vi "macro_TrajectoryConstraint_SwerveKine.vi"   [LabVIEW 2019, in "Trajectory_Library.lvlib"]
uses:
  Trajectory_Library.lvlib
types:
  T1 = typedef "WPILib_Math.lvlib/TRANSLATION2D.ctl" = cluster{"X":dbl, "Y":dbl}
  T2 = typedef "WPILib_Math.lvlib/SWERVE_DRIVE_KINEMATICS.ctl" = cluster{"NumModules":i32, "InverseKinematics":T3, "ForwardKinematics":T3, "Modules":T1[], "PrevCoR":T1, "SavedModuleStates":T4[]}
  T3 = typedef "NI_Matrix.lvlib/RealMatrix.ctl" = dbl[][]
  T4 = typedef "WPILib_Math.lvlib/SWERVE_DRIVE_MODULE_STATE.ctl" = cluster{"Speed":dbl, "Angle":T5}
  T5 = typedef "WPILib_Math.lvlib/ROTATION2D.ctl" = cluster{"VALUE":dbl, "COS":dbl, "SIN":dbl}
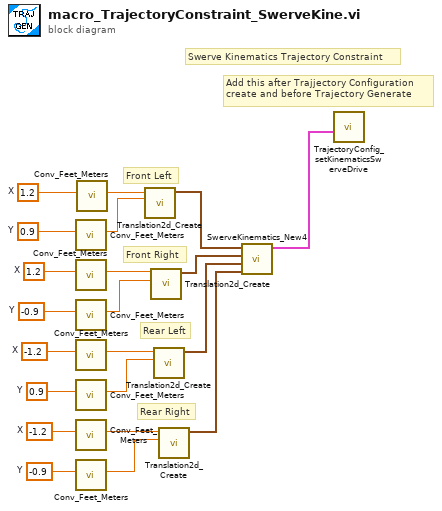
[diagram p0: block diagram]
diagram:
  w15 = -1.2  # X
  w14 = -0.9  # Y
  w17 = -1.2  # X
  w16 = 0.9  # Y
  w19 = 1.2  # X
  w18 = -0.9  # Y
  w21 = 1.2  # X
  w20 = 0.9  # Y
  # "Swerve Kinematics Trajectory Constraint"
  # "Rear Right"
  # "Rear Left"
  # "Front Right"
  # "Front Left"
  # "Add this after Trajjectory Configuration\ncreate and before Trajectory Generate"
  n1 = call "Conv_Feet_Meters.vi"("Feet"=w20) -> ("Meters"=w12:dbl)  [unwired: 10 in]
  n2 = call "Conv_Feet_Meters.vi"("Feet"=w19) -> ("Meters"=w11:dbl)  [unwired: 10 in]
  n3 = call "Conv_Feet_Meters.vi"("Feet"=w18) -> ("Meters"=w10:dbl)  [unwired: 10 in]
  n4 = call "Conv_Feet_Meters.vi"("Feet"=w17) -> ("Meters"=w9:dbl)  [unwired: 10 in]
  n5 = call "Conv_Feet_Meters.vi"("Feet"=w16) -> ("Meters"=w8:dbl)  [unwired: 10 in]
  n6 = call "Conv_Feet_Meters.vi"("Feet"=w15) -> ("Meters"=w7:dbl)  [unwired: 10 in]
  n7 = call "Conv_Feet_Meters.vi"("Feet"=w14) -> ("Meters"=w6:dbl)  [unwired: 10 in]
  n8 = call "Conv_Feet_Meters.vi"("Feet"=w21) -> ("Meters"=w13:dbl)  [unwired: 10 in]
  n9 = call "Translation2d_Create.vi"("Y"=w12, "X"=w13) -> ("TRANSLATION"=w4:T1)  [unwired: 9 in]
  n10 = call "Translation2d_Create.vi"("Y"=w10, "X"=w11) -> ("TRANSLATION"=w3:T1)  [unwired: 9 in]
  n11 = call "Translation2d_Create.vi"("Y"=w8, "X"=w9) -> ("TRANSLATION"=w2:T1)  [unwired: 9 in]
  n12 = call "Translation2d_Create.vi"("Y"=w6, "X"=w7) -> ("TRANSLATION"=w1:T1)  [unwired: 9 in]
  n13 = call "SwerveKinematics_New4.vi"("wheel 3"=w1, "wheel 2"=w2, "wheel 1"=w3, "wheel 0"=w4) -> ("SWERVE_DRIVE_KINEMATICS"=w5:T2)  [unwired: 7 in]
  n14 = call "TrajectoryConfig_setKinematicsSwerveDrive.vi"("SWERVE_DRIVE_KINEMATICS"=w5) -> ()  [unwired: 10 in, 1 out]
